vi "MotionStop.vi"(8 "error in (no error)":errorcluster, 10 "Quickcheck":bool, 11 "Tapedrive_ESP301 in":refnum<class "Tapedrive_ESP301.lvclass">) -> (0 "error out":errorcluster, 2 "new command":string, 3 "Tapedrive_ESP301 out":refnum<class "Tapedrive_ESP301.lvclass">)   [LabVIEW 2013, in "Tapedrive_ESP301.lvclass"]
uses:
  Tapedrive_ESP301.lvclass
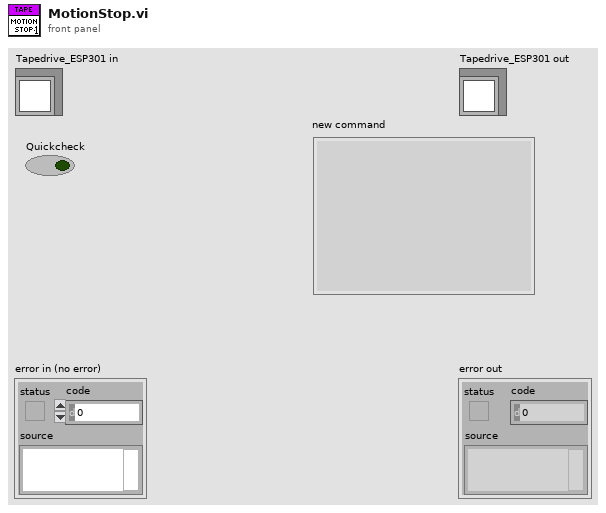
[diagram p1: front panel]
types:
  T1 = typedef "OnOffTypeDef.ctl" = enum16{"off", "on"}
  T2 = typedef "Direction.ctl" = enum16{"Forward", "Backward", "Undefined"}
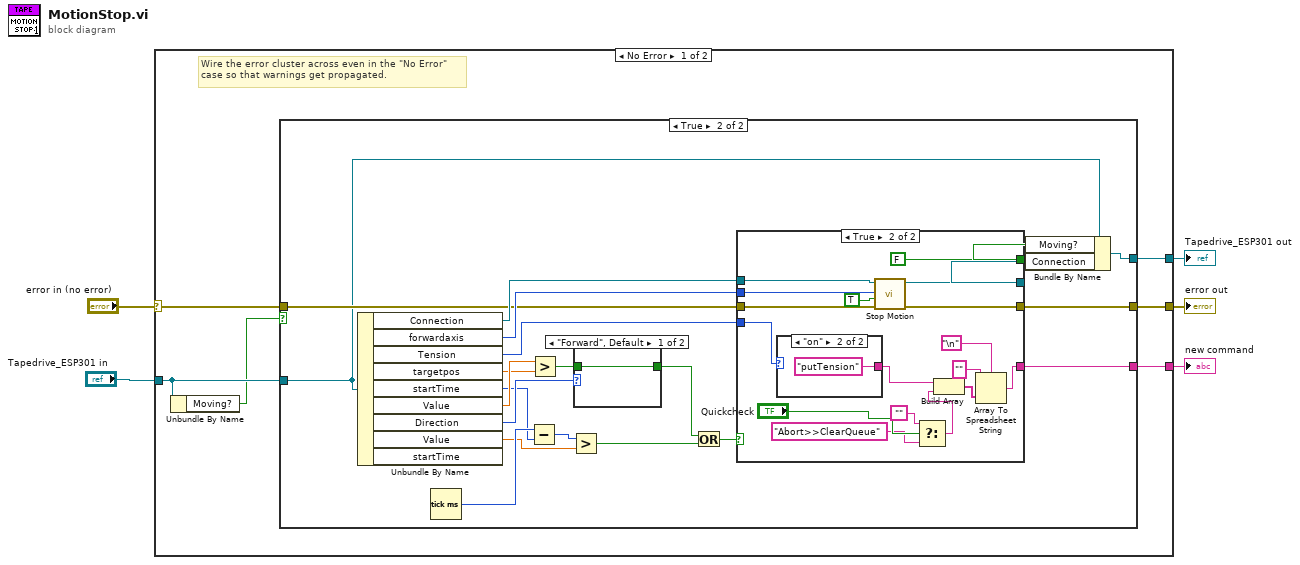
[diagram p0: block diagram]
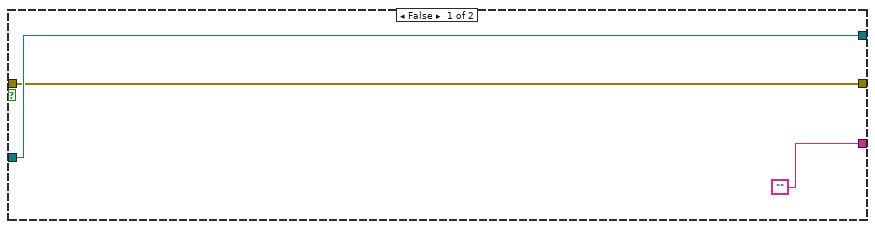
[diagram p2: hidden frame]
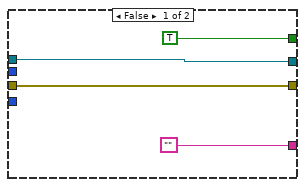
[diagram p3: hidden frame]
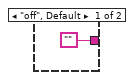
[diagram p4: hidden frame]
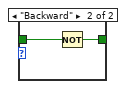
[diagram p5: hidden frame]
diagram:
  n1 = case shown="No Error" "error in (no error)" {
    selector: "error in (no error)" -> [w9 w63]
    tunnel: [w10 w63] -> w4
    tunnel: [w11 w62] -> w2
    tunnel: "Tapedrive_ESP301 in" -> [w7 w62]
    tunnel: [w8 _] -> w1
    frame No Error {
      # "Wire the error cluster across even in the \"No Error\"\ncase so that warnings get propagated."
      n2 = Unbundle By Name(w7) -> ("Moving?"=w6:bool)
      n3 = case shown="True" w6 {
        tunnel: [w14 w21] -> w11
        tunnel: [w13 w19] -> w10
        tunnel: w9 -> [w13 w18]
        tunnel: ["" w17] -> w8
        tunnel: w7 -> [w14 w15]
        frame False {
        }
        frame True {
          n4 = Unbundle By Name(w15) -> ("Connection"=w22:refnum<visa-resource-name>, "forwardaxis"=w23:i16, "Tension"=w24:T1, "targetpos"=w34:dbl, "startTime"=w30:u32, "Value"=w35:dbl, "Direction"=w33:T2, "Value"=w28:dbl)  [unwired: 1 out]
          n5 = Tick Count (ms)() -> (millisecond timer value=w31:u32)
          n6 = Subtract(x=w31, y=w30) -> (x-y=w29:u32)
          n7 = Greater?(x=w35, y=w34) -> (0:w32:bool)
          n8 = Greater?(x=w29, y=w28) -> (0:w27:bool)
          n9 = case shown="\"Forward\", Default" w33 {
            tunnel: [w59 w60] -> w26
            tunnel: w32 -> [w59 w61]
            frame "Forward", Default {
            }
            frame "Backward" {
              n10 = Not(x=w61) -> (.not. x?=w60:bool)
            }
          }
          n11 = Or(x=w26, y=w27) -> (x .or. y?=w25:bool)
          n12 = case shown="True" w25 {
            tunnel: w24 -> [_ w56]
            tunnel: w23 -> [_ w55]
            tunnel: w22 -> [w39 w54]
            tunnel: w18 -> [w38 w53]
            tunnel: [w38 w49] -> w19
            tunnel: [w39 w50] -> w16
            tunnel: ["" w40] -> w17
            tunnel: [TRUE ("Wait for Step") FALSE ("Wait for Step")] -> w20
            frame False {
            }
            frame True {
              n13 = case shown="\"on\"" w56 {
                tunnel: ["" "putTension"] -> w45
                frame "off", Default {
                }
                frame "on" {
                }
              }
              n14 = call <instrlib>:"Stop Motion.vi"("error in (no error)"=w53, "Stop all axes (F)"=TRUE, "Axis (1)"=w55, "VISA resource name"=w54) -> ("error out"=w49:errorcluster, "VISA resource name out"=w50:refnum<visa-resource-name>)  [unwired: 2 in]
              n15 = Select(t="", s="Quickcheck", f="Abort>>ClearQueue" ("string")) -> (s? t:f=w44:string)
              n16 = Build Array(w45, w44) -> (w43:string[])
              n17 = Array To Spreadsheet String(delimiter (Tab)="\n", array=w43, 3:"" ("format string")) -> (spreadsheet string=w40:string)
            }
          }
          n18 = Bundle By Name(cluster=w15, "Moving?"=w20, "Connection"=w16) -> (w21:refnum<class "Tapedrive_ESP301.lvclass">)
        }
      }
    }
    frame Error {
    }
  }
  "error out" <- w4
  "Tapedrive_ESP301 out" <- w2
  "new command" <- w1
